vi "Long Term PLot.vi"(0 "Graph Data":T1(array[cluster]), 5 "Plot Data":dbl[](array[numeric]), 9 "Clear Graph":bool, 11 "Max Number of Datapoints":dbl=10.0 format="%#_13g") -> (4 "Graph Data 2":T1(array[cluster]))   [LabVIEW 2020]
doc: "This VI plots data on xy graph and sets properties for xy graph\n[input]\n1. xy graph reference\n2. plot data\n3. graph array\n4. selected variables\n5. clear graph\n6. maximum no of points\n[output]\n1. xy plot"
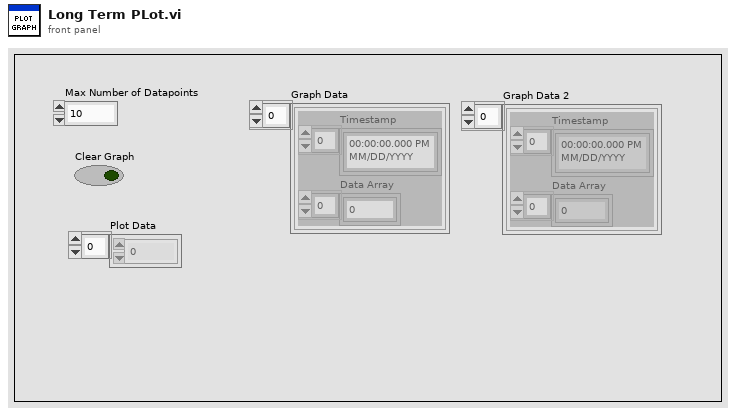
[diagram p1: front panel]
types:
  T1 = cluster{"Timestamp":timestamp[], "Data Array":dbl[]}[]
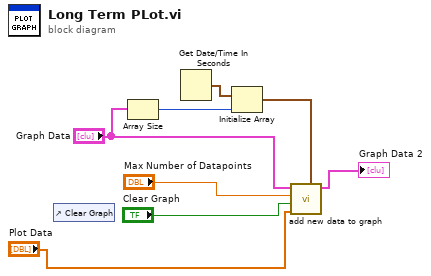
[diagram p0: block diagram]
diagram:
  n1 = control-ref of="Clear Graph"() -> ()  [unwired: 1 out]
  n2 = Array Size(array="Graph Data") -> (size(s)=w7:i32)
  n3 = Get Date/Time In Seconds() -> (seconds since 1Jan1904=w8:timestamp)
  n4 = Initialize Array(w8, w7) -> (w1:timestamp[])
  n5 = call "add new data to graph.vi"("New Timestamps"=w1, "Data Array"="Plot Data", "Clear Graph"="Clear Graph", "Max Number of Datapoints"="Max Number of Datapoints", "Graph Data"="Graph Data") -> ("Graph Data 2"=→"Graph Data 2":T1)  [unwired: 5 in]
